vi "Load JSON.vi"(6 "Expand all?":bool, 8 "Error In":errorcluster, 9 "JSON Schema in":string, 10 "<JSON> in":string, 11 "Component.JSONEditor in":refnum<class "Component.JSONEditor.lvclass">) -> (0 "Error Out":errorcluster, 3 "Component.JSONEditor out":refnum<class "Component.JSONEditor.lvclass">)   [LabVIEW 2021, in "Component.JSONEditor.lvclass"]
uses:
  Component.JSONEditor.lvclass
  E:/Git/WebView-Components/Source/Component_class/Component.lvclass
  <vilib>/JDP Science/JSONtext/LVClass Serializer/JSONtext LVClass Serializer.lvclass
  <vilib>/sklein/WebView2/Webview2 Lib/WebView2 Control Object/WebView2 Control.lvclass
  Editor Mode--enum.ctl
  40ff2670-f8ea-4d41-9900-15e563433872.vi
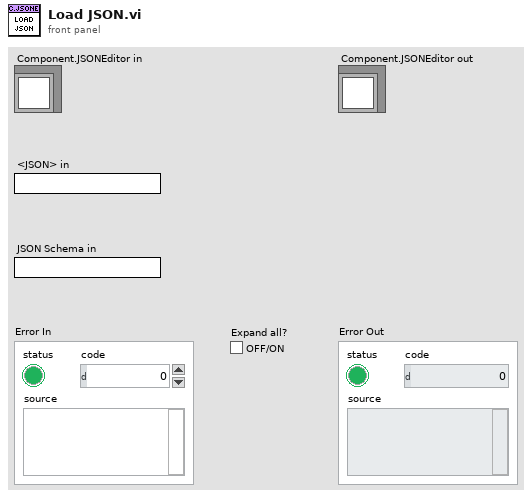
[diagram p1: front panel]
types:
  T1 = typedef "Component.JSONEditor.lvclass/Editor Mode--enum.ctl" = enum16{"Tree", "View", "Form", "Code", "Text"}
  T2 = cluster{"type":enum16{"loadJSON", "setMode", "getJSON"}, "json":string, "schema":string, "Mode":T1, "expandAll":bool}
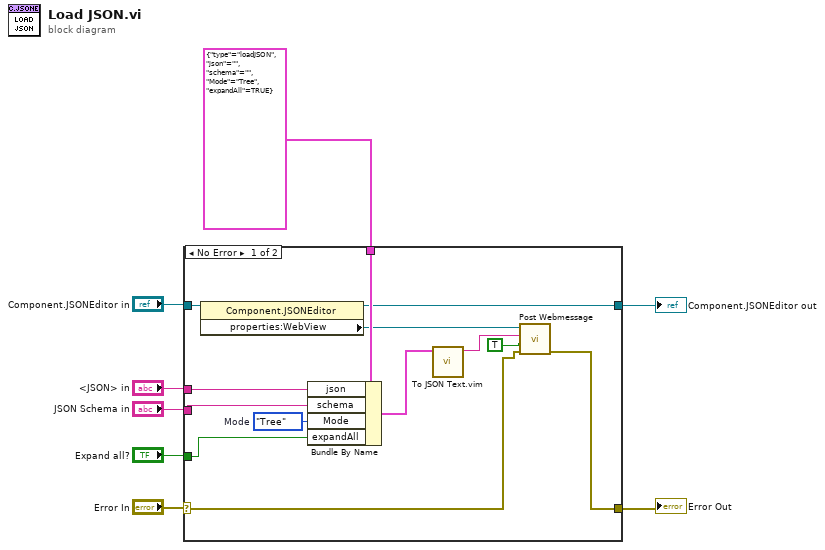
[diagram p0: block diagram]
diagram:
  n1 = case shown="No Error" "Error In" {
    selector: "Error In" -> [w11 w23]
    tunnel: [w10 w23] -> w7
    tunnel: [w9 w22] -> w5
    tunnel: "Component.JSONEditor in" -> [w15 w22]
    tunnel: "Expand all?" -> [w17 _]
    tunnel: "JSON Schema in" -> [w19 _]
    tunnel: "<JSON> in" -> [w20 _]
    tunnel: T2 {"type"=enum."loadJSON", "json"="", "schema"="", "Mode"=enum."Tree", "expandAll"=TRUE} -> [w21 _]
    frame No Error {
      w18 = Editor_Mode--enum."Tree"  # Mode
      n2 = property class="Component.JSONEditor"(reference=w15) -> (reference out=w9:refnum<class "Component.JSONEditor.lvclass">, "properties:WebView"=w14:refnum<class "WebView2 Control.lvclass">)  [unwired: 1 in, 1 out]
      n3 = Bundle By Name(cluster=w21, "json"=w20, "schema"=w19, "Mode"=w18, "expandAll"=w17) -> (w16:T2)
      n4 = call "To JSON Text.vim"("Anything"=w16) -> ("<JSON>"=w13:string)  [unwired: 9 in, 1 out]
      n5 = call <vilib>:"Post Webmessage.vi"("error in (no error)"=w11, "Send as JSON"=TRUE, "Message"=w13, "WebView2 Control in"=w14) -> ("error out"=w10:errorcluster)  [unwired: 6 in, 1 out]
    }
    frame Error {
    }
  }
  "Error Out" <- w7
  "Component.JSONEditor out" <- w5
